vi "Add RPTID.vi"(8 "error in (no error)":errorcluster, 11 "RPTID Data In":T1[](array[typedef])) -> (0 "error out":errorcluster)   [LabVIEW 2020, in "SECS Communication.lvlib" / "SECS Data Class.lvclass"]
uses:
  SECS Data Class.lvclass
  RPTID Data.ctl
  SECS Data Class.lvclass/SECS Data Class.ctl
  Get All RPTID Data.vi
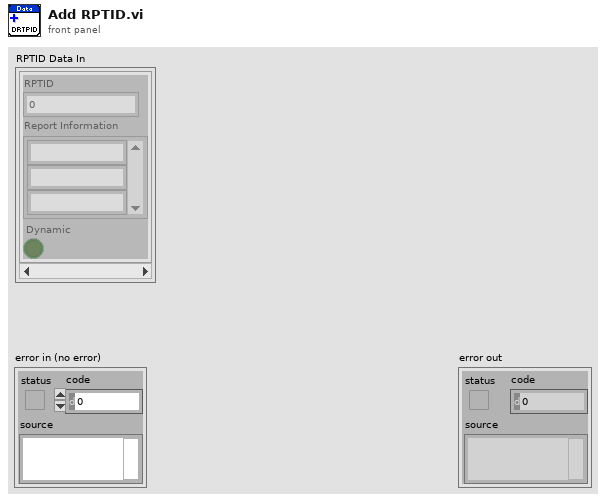
[diagram p1: front panel]
types:
  T1 = typedef "SECS Communication.lvlib/SECS Data Class.lvclass/RPTID Data.ctl" = cluster{"RPTID":u32, "Report Information":string[], "Dynamic":bool}
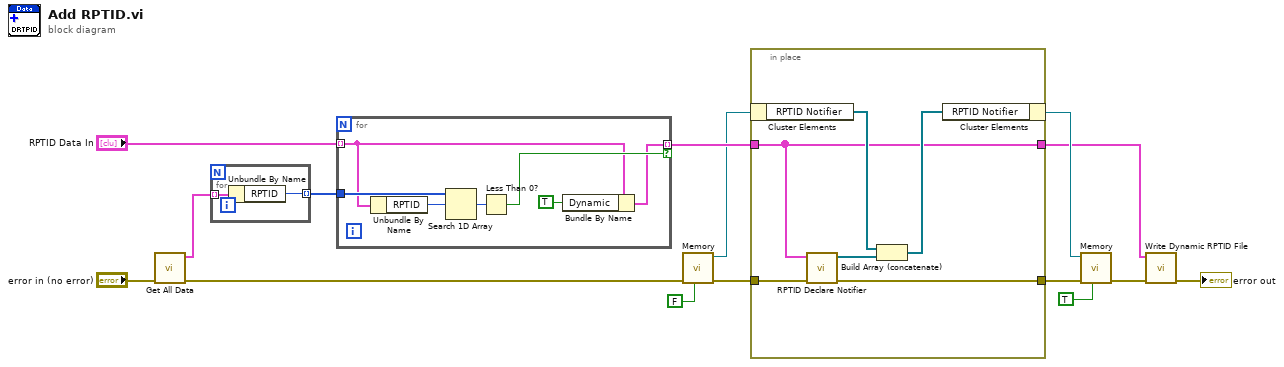
[diagram p0: block diagram]
diagram:
  n1 = call-poly "Get All Data.vi"("error in (no error)"="error in (no error)") -> ("error out"=w10:errorcluster, "RPTID Data"=w14:T1[])  [unwired: 9 in]
  n2 = for {
    tunnel: w14 -> [w17] mode=indexing
    tunnel: [w16] -> w13 mode=indexing
    n3 = Unbundle By Name(w17) -> ("RPTID"=w16:u32)
  }
  n4 = for {
    tunnel: w13 -> [w23]
    tunnel: "RPTID Data In" -> [w20] mode=indexing
    tunnel: [w18] -> w11 mode=indexing if=w21
    n5 = Unbundle By Name(w20) -> ("RPTID"=w22:u32)
    n6 = Search 1D Array(1D array=w23, element=w22) -> (index of element=w24:i32)  [unwired: 1 in]
    n7 = Less Than 0?(x=w24) -> (x < 0?=w21:bool)
    n8 = Bundle By Name(cluster=w20, "Dynamic"=TRUE) -> (w18:T1)
  }
  n9 = call "Memory.vi"("Put"=FALSE, "error in (no error)"=w10) -> ("error out"=w7:errorcluster, "SECS Data Class out"=w8:refnum<class "SECS Data Class.lvclass">)  [unwired: 8 in]
  n10 = in-place {
    in-place-border: w11 -> [w25]
    in-place-border: w7 -> [w30]
    in-place-border: [w26] -> w6
    in-place-border: [w25] -> w2
    n11 = in-place-cluster #1(w8) -> ("RPTID Notifier"=w28:refnum<notifier>[])
    n12 = call "RPTID Declare Notifier.vi"("error in"=w30, "RPTID Data"=w25) -> ("error out"=w26:errorcluster, "RPTID Notifier"=w29:refnum<notifier>[])  [unwired: 8 in]
    n13 = Build Array (concatenate)(w28, w29) -> (w27:refnum<notifier>[])
    n14 = in-place-cluster #1("RPTID Notifier"=w27) -> (w5:refnum<class "SECS Data Class.lvclass">)
  }
  n15 = call "Memory.vi"("Put"=TRUE, "error in (no error)"=w6, "SECS Data Class in"=w5) -> ("error out"=w3:errorcluster)  [unwired: 7 in, 1 out]
  n16 = call "Write Dynamic RPTID File.vi"("error in (no error)"=w3, "RPTID Data In"=w2) -> ("error out"=→"error out":errorcluster)  [unwired: 9 in]
